vi "Store Actor Core Ref.vi"(8 "error in (no error)":errorcluster, 11 "IViewable In":refnum<class "IViewable.lvclass">) -> (0 "error out":errorcluster, 3 "IViewable Out":refnum<class "IViewable.lvclass">)   [LabVIEW 2015, in "IViewable.lvlib" / "IViewable.lvclass"]
uses:
  IViewable.lvclass
  IViewable.lvclass/IViewable.ctl
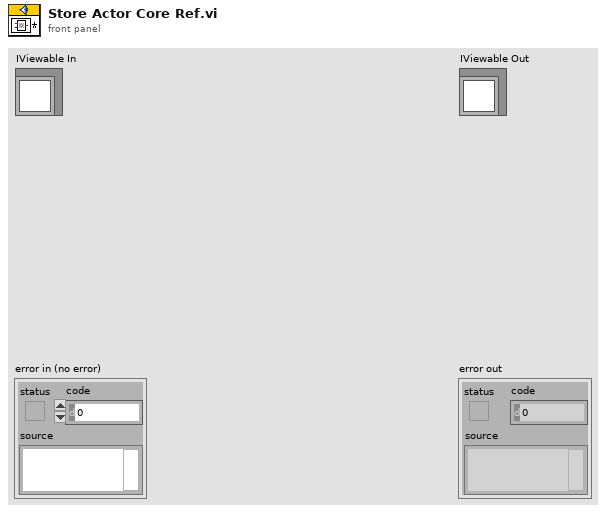
[diagram p1: front panel]
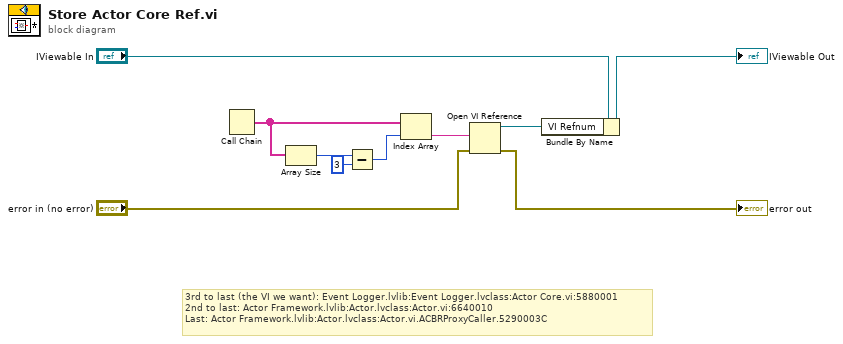
[diagram p0: block diagram]
diagram:
  # "3rd to last (the VI we want): Event Logger.lvlib:Event Logger.lvclass:Actor Core.vi:5880001\n2nd to last: Actor Framework.lvlib:Actor.lvclass:Actor.vi:6640010\nLast: Actor Framework.lvlib:Actor.lvclass:Actor.vi.ACBRProxyCaller.5290003C"
  n1 = Call Chain() -> (call chain=w4:string[])
  n2 = Array Size(array=w4) -> (size(s)=w6:i32)
  n3 = Subtract(x=w6, y=3) -> (x-y=w3:i32)
  n4 = Index Array(array=w4, index=w3) -> (element=w1:string)
  n5 = Open VI Reference(vi path=w1, error in (no error)="error in (no error)") -> (vi reference=w2:refnum<vi>, error out=→"error out":errorcluster)  [unwired: 4 in]
  n6 = Bundle By Name(cluster="IViewable In", "VI Refnum"=w2) -> (→"IViewable Out":refnum<class "IViewable.lvclass">)
